vi "Chat_main - subvi_ver.vi"() -> ()   [LabVIEW 2012]
uses:
  Controls/Stage.ctl
panel:
  in  "Port":u16=13078
  in  "Host IP":string="127.0.0.1"
  out "OnlineList":string[](array[string])
  in  "Create":bool
  in  "OffLine":bool
  in  "Link":bool
  out "linked":bool
  in  "Nickname":string
  in  "Send":bool
  in  "MsgBox":string
  out "C_Room":string
  # "sub ver"
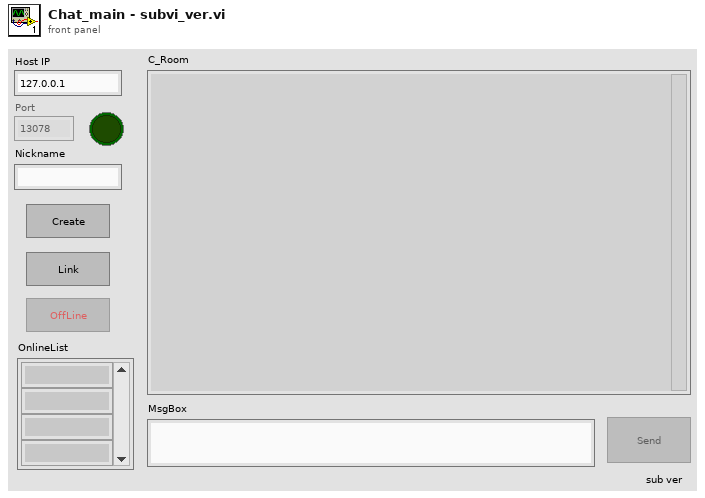
[diagram p1: front panel]
types:
  T1 = typedef "Stage.ctl" = enum16{"Initial", "Idle", "Link", "TX", "RX", "stop"}
  T2 = enum8{"Enabled", "Disabled", "Disabled and Grayed Out"}
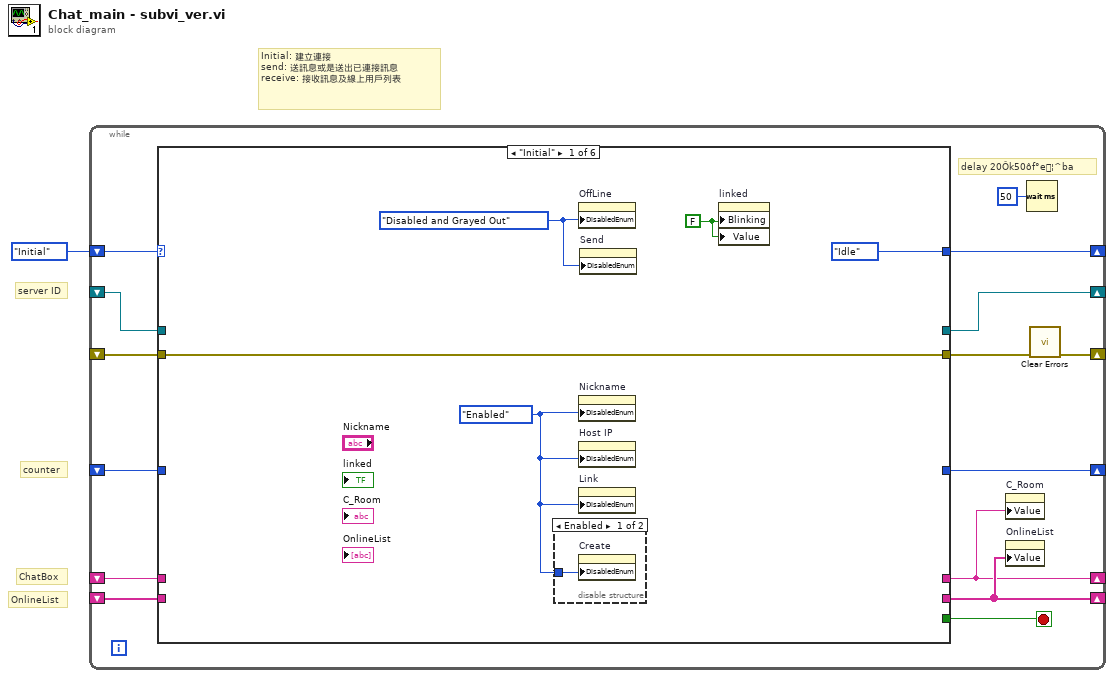
[diagram p0: block diagram]
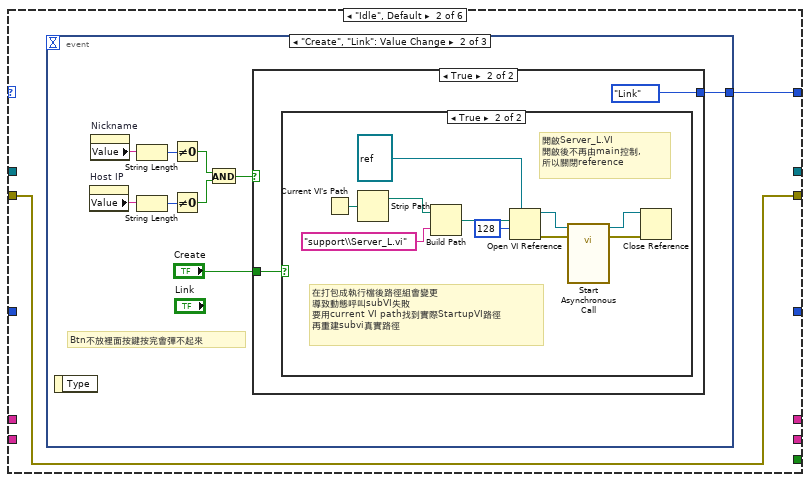
[diagram p3: hidden frame]
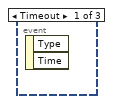
[diagram p4: hidden frame]
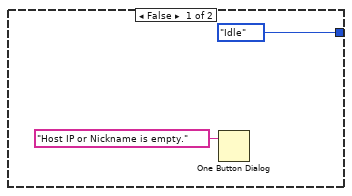
[diagram p5: hidden frame]
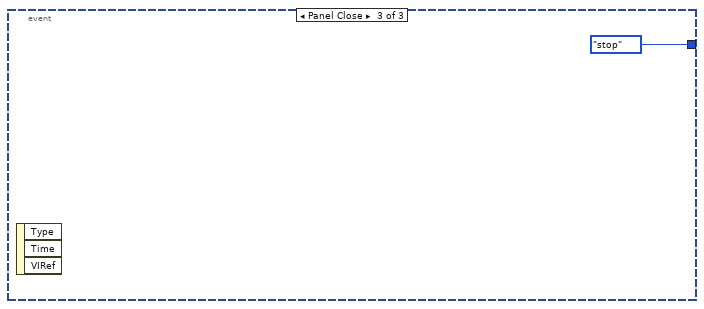
[diagram p7: hidden frame]
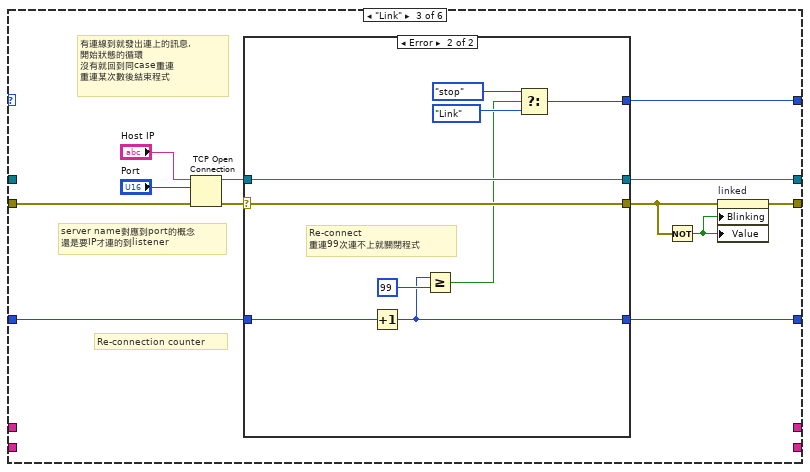
[diagram p8: hidden frame]
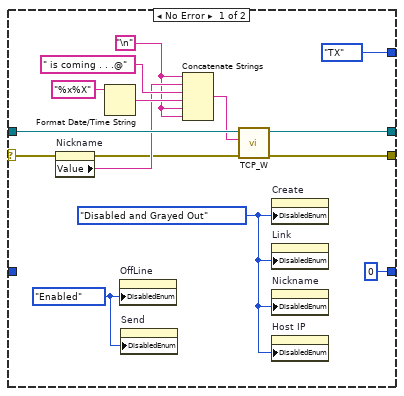
[diagram p9: hidden frame]
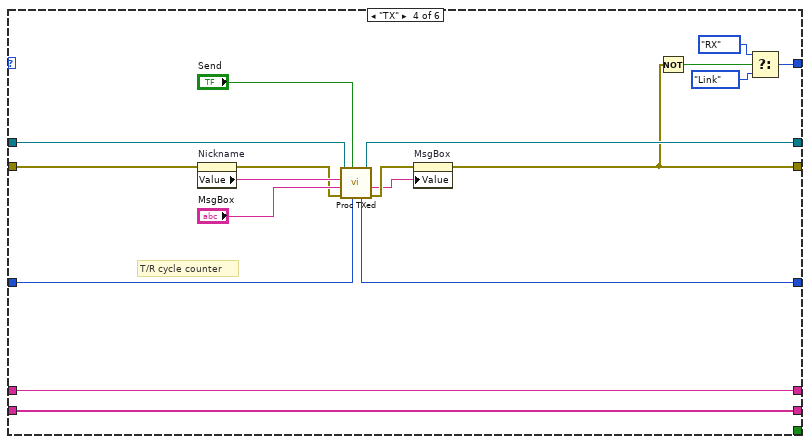
[diagram p10: hidden frame]
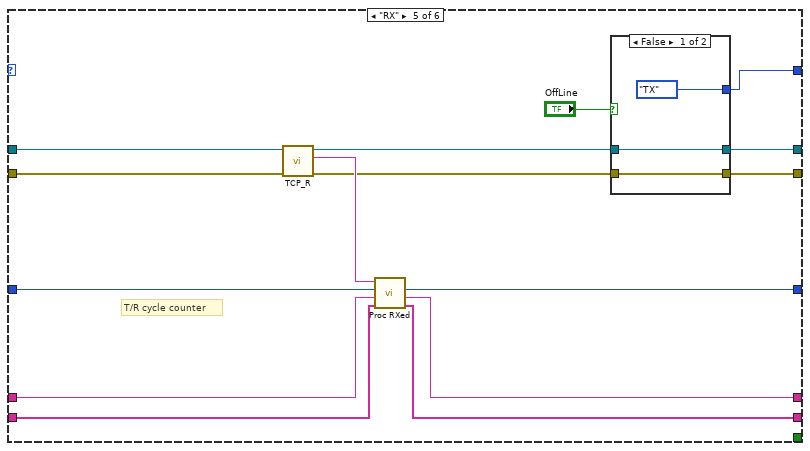
[diagram p11: hidden frame]
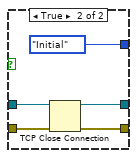
[diagram p12: hidden frame]
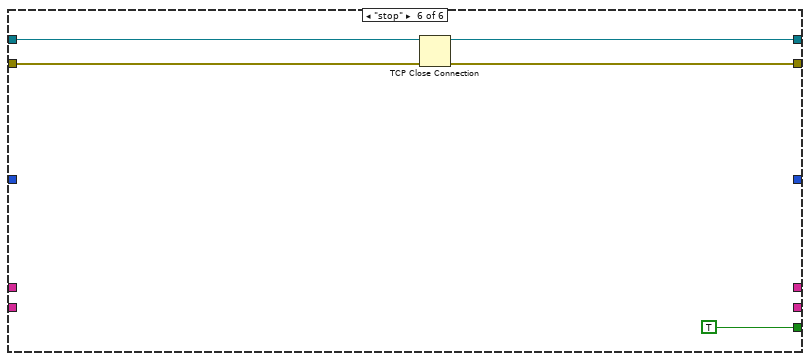
[diagram p13: hidden frame]
diagram:
  # "OnlineList"
  # "ChatBox"
  # "server ID"
  # "counter"
  # "Initial: 建立連接\nsend: 送訊息或是送出已連接訊息\nreceive: 接收訊息及線上用戶列表"
  n1 = while {
    shift-right: [w15] -> _
    shift-left: Stage."Initial" -> [w16]
    shift-right: [w13] -> _
    shift-left: _ -> [w12]
    shift-right: [w6] -> _
    shift-left: _ -> [w11]
    shift-right: [w8] -> _
    shift-left: _ -> [w9]
    shift-right: [w2] -> _
    shift-left: _ -> [w3]
    shift-right: [w5] -> _
    shift-left: _ -> [w4]
    stop <- w14 stop-if-true
    # "delay 20Ôk50ôf°e¦^ba"
    n2 = case shown="\"Initial\"" w16 {
      tunnel: [Stage."Idle" w24 w57 w98 w112 _] -> w15
      tunnel: [_ _ _ _ _ TRUE ("stop")] -> w14
      tunnel: [_ _ w59 w101 w113 w126] -> w13
      tunnel: w12 -> [_ _ _ w102 w117 w129]
      tunnel: [w18 w23 w49 w91 w111 w128] -> w7
      tunnel: w11 -> [w18 w23 w53 w89 w116 w127]
      tunnel: w9 -> [_ _ w56 w86 w110 _]
      tunnel: [_ _ w55 w87 w106 _] -> w8
      tunnel: [_ _ _ w94 w104 _] -> w5
      tunnel: w4 -> [_ _ _ w94 w105 _]
      tunnel: w3 -> [_ _ _ w95 w107 _]
      tunnel: [_ _ _ w95 w103 _] -> w2
      frame "Initial" {
        w17 = T2."Enabled" ("Disabled")
        w19 = FALSE ("Link")
        w20 = T2."Disabled and Grayed Out" ("Disabled")
        n3 = disable-structure shown="Enabled" {
          disable-tunnel: w17 -> [w22 _]
          frame Enabled {
            n4 = property on="Create" class="Bool"("DisabledEnum"=w22) -> ()  [unwired: 2 in, 2 out]
          }
          frame Disabled {
          }
        }
        n5 = property on="OffLine" class="Bool"("DisabledEnum"=w20) -> ()  [unwired: 2 in, 2 out]
        n6 = property on="Nickname" class="Str"("DisabledEnum"=w17) -> ()  [unwired: 2 in, 2 out]
        n7 = property on="Host IP" class="Str"("DisabledEnum"=w17) -> ()  [unwired: 2 in, 2 out]
        n8 = property on="Link" class="Bool"("DisabledEnum"=w17) -> ()  [unwired: 2 in, 2 out]
        n9 = property on="Send" class="Bool"("DisabledEnum"=w20) -> ()  [unwired: 2 in, 2 out]
        n10 = property on="linked" class="Bool (strict)"("Blinking"=w19, "Value"=w19) -> ()  [unwired: 2 in, 2 out]
      }
      frame "Idle", Default {
        n11 = event shown="[1] \"Create\", \"Link\": Value Change" {
          selector: _ -> [_ _ _]
          dyn-events: _ -> [_ _ _]
          timeout: _ -> [_ _ _]
          tunnel: [_ w33 Stage."stop"] -> w24
          event Timeout {
            n12 = event-data() -> ()  [unwired: 1 in, 2 out]
          }
          event "Create", "Link": Value Change {
            # "Btn不放裡面按鍵按完會彈不起來"
            n13 = event-data() -> ()  [unwired: 1 in, 1 out]
            n14 = property on="Host IP" class="Str"() -> ("Value"=w26:string)  [unwired: 2 in, 2 out]
            n15 = property on="Nickname" class="Str"() -> ("Value"=w29:string)  [unwired: 2 in, 2 out]
            n16 = String Length(string=w29) -> (length=w32:i32)
            n17 = String Length(string=w26) -> (length=w30:i32)
            n18 = Not Equal To 0?(x=w32) -> (x != 0?=w28:bool)
            n19 = Not Equal To 0?(x=w30) -> (x != 0?=w27:bool)
            n20 = And(x=w28, y=w27) -> (x .and. y?=w31:bool)
            n21 = case shown="True" w31 {
              tunnel: [Stage."Idle" Stage."Link"] -> w33
              tunnel: "Create" -> [_ w36]
              frame False {
                n22 = One Button Dialog(message="Host IP or Nickname is empty.") -> ()  [unwired: 1 in, 1 out]
              }
              frame True {
                n23 = case shown="True" w36 {
                  frame False {
                  }
                  frame True {
                    # "在打包成執行檔後路徑組會變更\n導致動態呼叫subVI失敗\n要用current VI path找到實際StartupVI路徑\n再重建subvi真實路徑"
                    # "開啟Server_L.VI\n開啟後不再由main控制,\n所以關閉reference"
                    n24 = Current VI's Path() -> (path=w39:path)
                    n25 = Strip Path(path=w39) -> (stripped path=w38:path)  [unwired: 1 out]
                    n26 = Build Path(base path=w38, name or relative path="support\\Server_L.vi" ("vi path")) -> (appended path=w43:path)
                    n27 = Open VI Reference(type specifier VI Refnum (for type only)=refnum<vi> refnum, vi path=w43, options=128) -> (vi reference=w47:refnum<vi>, error out=w45:errorcluster)  [unwired: 3 in]
                    n28 = call-by-ref "Start Asynchronous Call"(reference=w47, error in=w45) -> (reference out=w40:refnum<vi>, error out=w41:errorcluster)  [unwired: 12 in]
                    n29 = Close Reference(reference=w40, error in (no error)=w41) -> ()  [unwired: 1 out]
                  }
                }
              }
            }
          }
          event Panel Close {
            n30 = event-data() -> ()  [unwired: 1 in, 3 out]
          }
        }
      }
      frame "Link" {
        # "Re-connection counter"
        # "server name對應到port的概念\n還是要IP才連的到listener"
        # "有連線到就發出連上的訊息,\n開始狀態的循環\n沒有就回到同case重連\n重連某次數後結束程式"
        n31 = TCP Open Connection(address="Host IP", remote port or service name="Port", error in (no error)=w53) -> (connection ID=w60:refnum<k5>, error out=w58:errorcluster)  [unwired: 2 in]
        n32 = case shown="Error" w58 {
          selector: w58 -> [w62 w83]
          tunnel: [w65 w83] -> w50
          tunnel: w60 -> [w75 w84]
          tunnel: [w66 w84] -> w59
          tunnel: [Stage."TX" w81] -> w57
          tunnel: w56 -> [_ w82]
          tunnel: [0 w77] -> w55
          frame No Error {
            w64 = T2."Disabled and Grayed Out" ("Disabled")
            w67 = T2."Enabled" ("Disabled")
            w63 = "\n"
            n33 = property on="Nickname" class="Str"(error in=w62) -> (error out=w61:errorcluster, "Value"=w68:string)  [unwired: 1 in, 1 out]
            n34 = Format Date/Time String(time format string (%c)="%x%X") -> (date/time string=w69:string)  [unwired: 2 in]
            n35 = property on="OffLine" class="Bool"("DisabledEnum"=w67) -> ()  [unwired: 2 in, 2 out]
            n36 = property on="Send" class="Bool"("DisabledEnum"=w67) -> ()  [unwired: 2 in, 2 out]
            n37 = Concatenate Strings(w63, w68, " is coming . . .@" ("data in"), w69, w63, w63) -> (w71:string)
            n38 = call "TCP_W.vi"("error in"=w61, "data in"=w71, "connection ID"=w75) -> ("error IO"=w65:errorcluster, "connection ID out"=w66:refnum<k5>)  [unwired: 7 in]
            n39 = property on="Create" class="Bool"("DisabledEnum"=w64) -> ()  [unwired: 2 in, 2 out]
            n40 = property on="Link" class="Bool"("DisabledEnum"=w64) -> ()  [unwired: 2 in, 2 out]
            n41 = property on="Nickname" class="Str"("DisabledEnum"=w64) -> ()  [unwired: 2 in, 2 out]
            n42 = property on="Host IP" class="Str"("DisabledEnum"=w64) -> ()  [unwired: 2 in, 2 out]
          }
          frame Error {
            # "Re-connect\n重連99次連不上就關閉程式"
            n43 = Increment(x=w82) -> (x+1=w77:i32)
            n44 = Greater Or Equal?(x=w77, y=99) -> (x >= y?=w76:bool)
            n45 = Select(t=Stage."stop", s=w76, f=Stage."Link") -> (s? t:f=w81:T1)
          }
        }
        n46 = Not(x=w50) -> (.not. x?=w54:bool)
        n47 = property on="linked" class="Bool (strict)"(error in=w50, "Blinking"=w54, "Value"=w54) -> (error out=w49:errorcluster)  [unwired: 1 in, 1 out]
      }
      frame "TX" {
        # "T/R cycle counter"
        n48 = property on="Nickname" class="Str"(error in=w89) -> (error out=w88:errorcluster, "Value"=w90:string)  [unwired: 1 in, 1 out]
        n49 = call "Proc TXed.vi"("counter in"=w86, "Send"="Send", "error in"=w88, "MsgBox in"="MsgBox", "Nickname"=w90, "Connection in"=w102) -> ("error out"=w92:errorcluster, "MsgBox out"=w85:string, "Connection out"=w101:refnum<k5>, "counter out"=w87:i32)  [unwired: 2 in]
        n50 = property on="MsgBox" class="Str"(error in=w92, "Value"=w85) -> (error out=w91:errorcluster)  [unwired: 1 in, 1 out]
        n51 = Not(x=w91) -> (.not. x?=w97:bool)
        n52 = Select(t=Stage."RX", s=w97, f=Stage."Link") -> (s? t:f=w98:T1)
      }
      frame "RX" {
        # "T/R cycle counter"
        n53 = call "TCP_R.vi"("error in"=w116, "connection ID"=w117) -> ("error out"=w108:errorcluster, "data out"=w109:string, "connection ID out"=w114:refnum<k5>)  [unwired: 7 in]
        n54 = call "Proc RXed.vi"("List in"=w105, "MsgBox in"=w107, "counter in"=w110, "data in"=w109) -> ("List out"=w104:string[], "MsgBox out"=w103:string, "counter out"=w106:i32)  [unwired: 5 in]
        n55 = case shown="False" "OffLine" {
          tunnel: [Stage."TX" Stage."Initial"] -> w112
          tunnel: w114 -> [w119 w124]
          tunnel: [w119 w123] -> w113
          tunnel: [w118 w122] -> w111
          tunnel: w108 -> [w118 w121]
          frame False {
          }
          frame True {
            n56 = TCP Close Connection(connection ID=w124, error in (no error)=w121) -> (connection ID out=w123:refnum<k5>, error out=w122:errorcluster)  [unwired: 1 in]
          }
        }
      }
      frame "stop" {
        n57 = TCP Close Connection(connection ID=w129, error in (no error)=w127) -> (connection ID out=w126:refnum<k5>, error out=w128:errorcluster)  [unwired: 1 in]
      }
    }
    n58 = property on="C_Room" class="Str"("Value"=w2) -> ()  [unwired: 2 in, 2 out]
    n59 = property on="OnlineList" class="Arr (strict)"("Value"=w5) -> ()  [unwired: 2 in, 2 out]
    n60 = Wait (ms)(milliseconds to wait=u32 50) -> ()  [unwired: 1 out]
    n61 = call <vilib>:"Clear Errors.vi"("error in (no error)"=w7) -> ("error out"=w6:errorcluster)  [unwired: 5 in, 1 out]
  }
